vi "channel separator.vi"() -> ()   [LabVIEW 2014]
panel:
  out "Array":i32[](array[numeric])
  out "output array":dbl[][](array[numeric])
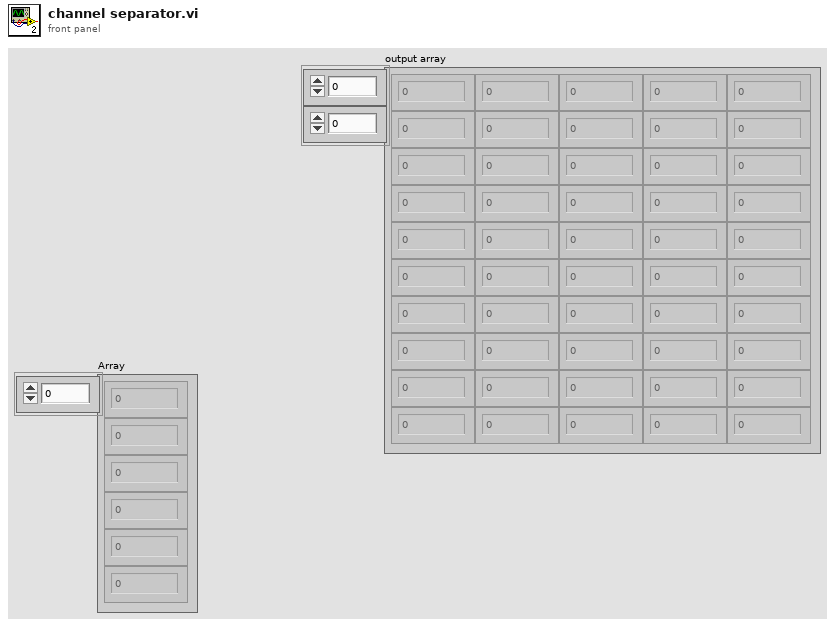
[diagram p1: front panel]
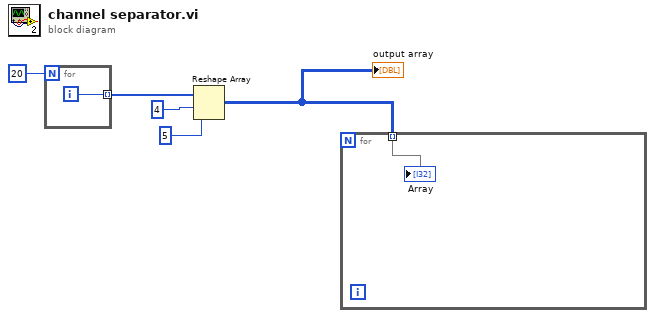
[diagram p0: block diagram]
diagram:
  n1 = for {
    N: 20 ("Numeric Control") -> [_]
    tunnel: [w6] -> w3 mode=indexing
    i -> [w6]
  }
  n2 = Reshape Array(w3, 4 ("dimension size"), 5 ("dimension size")) -> (w1:i32[][])
  "output array" <- w1
  n3 = for {
    tunnel: w1 -> [w7] mode=indexing
    "Array" <- w7
  }
